vi "Write Data.vi"(10 "Data":dbl[](array[numeric]), 11 "WT1600 in":refnum<class "WT1600.lvclass">) -> (3 "WT1600 out":refnum<class "WT1600.lvclass">)   [LabVIEW 2012, in "WT1600.lvlib" / "WT1600.lvclass"]
uses:
  WT1600.lvclass
  WT1600.lvclass/WT1600.ctl
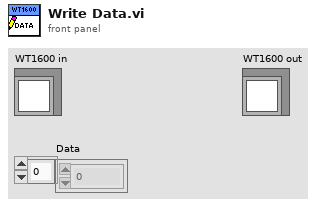
[diagram p1: front panel]
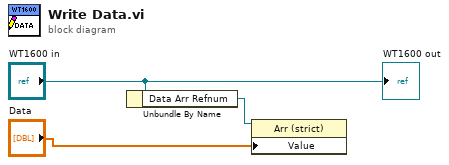
[diagram p0: block diagram]
diagram:
  n1 = Unbundle By Name("WT1600 in") -> ("Data Arr Refnum"=w2:refnum<vi>)
  n2 = property class="Arr (strict)"(reference=w2, "Value"="Data") -> ()  [unwired: 1 in, 2 out]
  "WT1600 out" <- "WT1600 in"
